vi "plant_write_checkpoint_spec.vi"(3 "Dataflow In":errorcluster) -> (1 "Dataflow Out":errorcluster)   [LabVIEW 2019]
uses:
  lib/libSimulationControl/libSimulationControl.lvlib
panel:
  out "Old Specification":path
  out "Working Directory":path
  out "New Specification":path
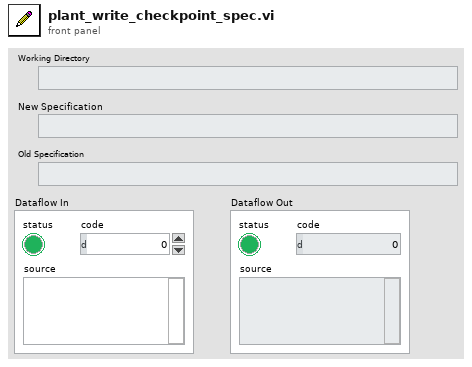
[diagram p1: front panel]
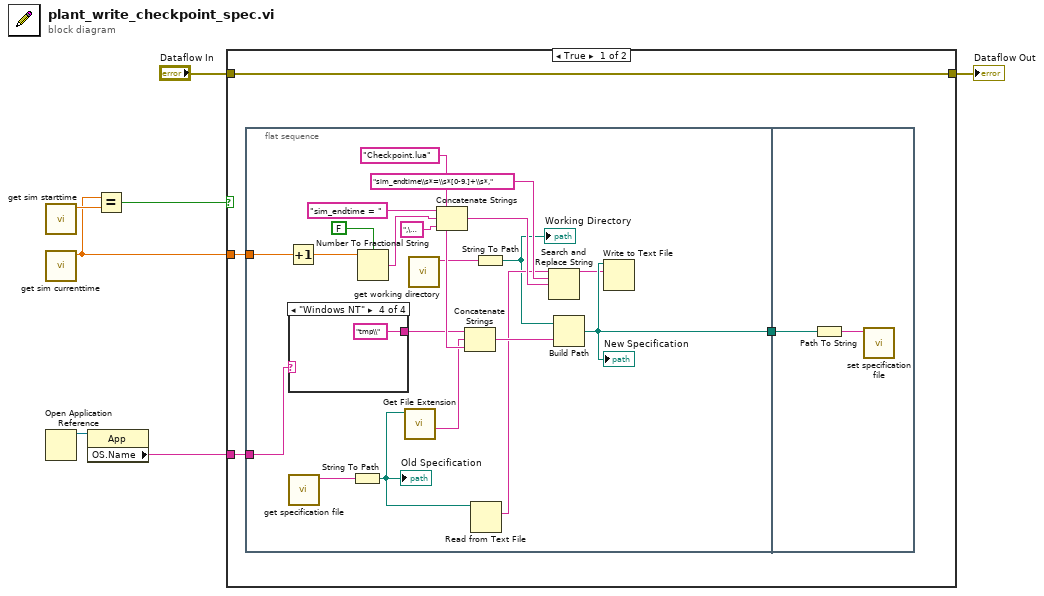
[diagram p0: block diagram]
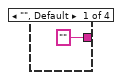
[diagram p2: hidden frame]
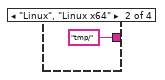
[diagram p3: hidden frame]
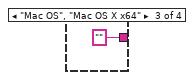
[diagram p4: hidden frame]
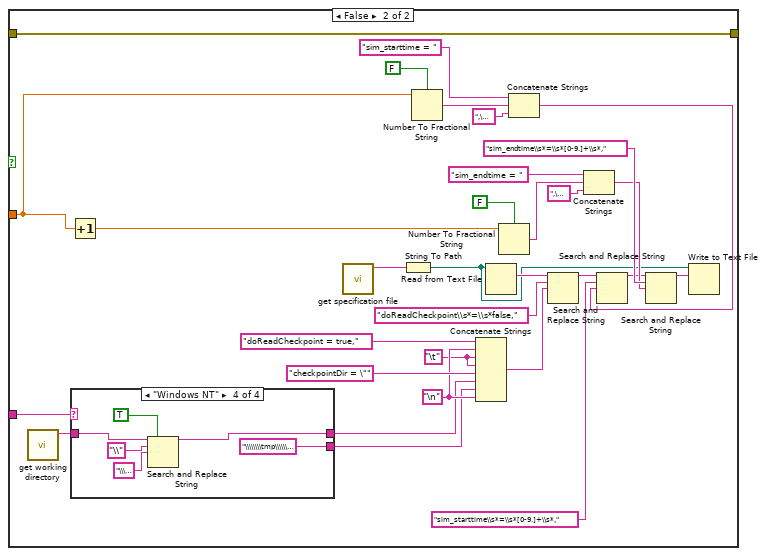
[diagram p5: hidden frame]
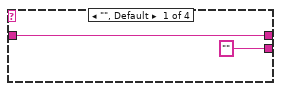
[diagram p6: hidden frame]
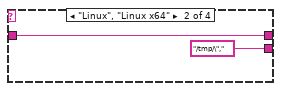
[diagram p7: hidden frame]
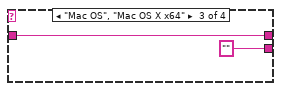
[diagram p8: hidden frame]
diagram:
  n1 = call "get sim starttime.vi"() -> ("function return"=w6:dbl)  [unwired: 10 in, 1 out]
  n2 = call "get sim currenttime.vi"() -> ("function return"=w5:dbl)  [unwired: 10 in, 1 out]
  n3 = Open Application Reference() -> (3:w4:refnum<vi>)  [unwired: 4 in, 1 out]
  n4 = property class="App"(reference=w4) -> ("OS.Name"=w3:string)  [unwired: 1 in, 2 out]
  n5 = Equal?(x=w5, y=w6) -> (x = y?=w7:bool)
  n6 = case shown="True" w7 {
    tunnel: w5 -> [w10 w68]
    tunnel: w3 -> [w9 w42]
    tunnel: [w8 w38] -> w2
    tunnel: "Dataflow In" -> [w8 w38]
    frame True {
      n7 = flat-sequence {
        tunnel: [w27] -> w11
        tunnel: w10 -> [w25]
        tunnel: w9 -> [w13]
        tunnel: w11 -> [w37]
        frame #0 {
          n8 = Increment(x=w25) -> (x+1=w18:dbl)
          n9 = case shown="\"Windows NT\"" w13 {
            tunnel: ["" ("return type") "tmp/" ("name or relative path") "" ("return type") "tmp\\" ("name or relative path")] -> w12
            frame "", Default {
            }
            frame "Linux", "Linux x64" {
            }
            frame "Mac OS", "Mac OS X x64" {
            }
            frame "Windows NT" {
            }
          }
          n10 = call "get specification file.vi"() -> ("function return"=w15:string)  [unwired: 10 in, 1 out]
          n11 = String To Path(string=w15) -> (path=w28:path)
          "Old Specification" <- w28
          n12 = Number To Fractional String(use system decimal point (T)=FALSE, number=w18) -> (F-format string=w23:string)  [unwired: 2 in]
          n13 = call <vilib>:"Get File Extension.vi"("file"=w28) -> ("filename without extension"=w29:string)  [unwired: 6 in, 4 out]
          n14 = call "get working directory.vi"() -> ("function return"=w14:string)  [unwired: 10 in, 1 out]
          n15 = Concatenate Strings("sim_endtime = " ("replace string (\"\")"), w23, ",\u0000\\n" ("string")) -> (w21:string)
          n16 = Concatenate Strings(w12, w29, "Checkpoint.lua" ("string")) -> (w30:string)
          n17 = Read from Text File(file (use dialog)=w28) -> (text=w17:string)  [unwired: 3 in, 3 out]
          n18 = String To Path(string=w14) -> (path=w16:path)
          "Working Directory" <- w16
          n19 = Search and Replace String(input string=w17, search string="sim_endtime\\s*=\\s*[0-9.]+\\s*,", replace string=w21) -> (result string=w20:string)  [unwired: 5 in, 3 out]
          n20 = Build Path(base path=w16, name or relative path=w30) -> (appended path=w27:path)
          "New Specification" <- w27
          n21 = Write to Text File(file (use dialog)=w27, text=w20) -> ()  [unwired: 2 in, 3 out]
        }
        frame #1 {
          n22 = Path To String(path=w37) -> (string=w36:string)
          n23 = call "set specification file.vi"("spec_file"=w36) -> ()  [unwired: 10 in, 1 out]
        }
      }
    }
    frame False {
      w61 = "\t"
      w62 = "\n"
      n24 = call "get working directory.vi"() -> ("function return"=w40:string)  [unwired: 10 in, 1 out]
      n25 = Increment(x=w68) -> (x+1=w67:dbl)
      n26 = case shown="\"Windows NT\"" w42 {
        tunnel: ["" ("return type") "/tmp/\"," ("name or relative path") "" ("return type") "\\\\\\\\tmp\\\\\\\\\"," ("name or relative path")] -> w41
        tunnel: w40 -> [w69 w71 w73 w76]
        tunnel: [w69 w71 w73 w75] -> w39
        frame "", Default {
        }
        frame "Linux", "Linux x64" {
        }
        frame "Mac OS", "Mac OS X x64" {
        }
        frame "Windows NT" {
          n27 = Search and Replace String(replace all?=TRUE ("Alle ersetzen? (F)"), input string=w76, search string="\\" ("Such-String"), replace string="\\\\\\\\" ("Ersetzungs-String (\"\")")) -> (result string=w75:string)  [unwired: 4 in, 3 out]
        }
      }
      n28 = call "get specification file.vi"() -> ("function return"=w43:string)  [unwired: 10 in, 1 out]
      n29 = String To Path(string=w43) -> (path=w44:path)
      n30 = Number To Fractional String(use system decimal point (T)=FALSE, number=w68) -> (F-format string=w57:string)  [unwired: 2 in]
      n31 = Concatenate Strings("doReadCheckpoint = true," ("search string"), w62, w61, w61, "checkpointDir = \"" ("string"), w39, w41, w62) -> (w64:string)
      n32 = Read from Text File(file (use dialog)=w44) -> (text=w45:string)  [unwired: 3 in, 3 out]
      n33 = Number To Fractional String(use system decimal point (T)=FALSE, number=w67) -> (F-format string=w52:string)  [unwired: 2 in]
      n34 = Concatenate Strings("sim_starttime = " ("replace string (\"\")"), w57, ",\u0000\\n" ("string")) -> (w59:string)
      n35 = Search and Replace String(input string=w45, search string="doReadCheckpoint\\s*=\\s*false,", replace string=w64) -> (result string=w55:string)  [unwired: 5 in, 3 out]
      n36 = Concatenate Strings("sim_endtime = " ("replace string (\"\")"), w52, ",\u0000\\n" ("string")) -> (w50:string)
      n37 = Search and Replace String(input string=w55, search string="sim_starttime\\s*=\\s*[0-9.]+\\s*,", replace string=w59) -> (result string=w49:string)  [unwired: 5 in, 3 out]
      n38 = Search and Replace String(input string=w49, search string="sim_endtime\\s*=\\s*[0-9.]+\\s*,", replace string=w50) -> (result string=w48:string)  [unwired: 5 in, 3 out]
      n39 = Write to Text File(file (use dialog)=w44, text=w48) -> ()  [unwired: 2 in, 3 out]
    }
  }
  "Dataflow Out" <- w2
